vi "Core Actor - CLOSE - External Queues_Notifiers.vi"(8 "error in (no error)":errorcluster, 11 "Child_4_Class in":refnum<class "Logging_Class.lvclass">) -> (0 "error out":errorcluster, 3 "Child_4_Class out":refnum<class "Logging_Class.lvclass">)   [LabVIEW 2023, in "Logging.lvlib" / "Logging_Class.lvclass"]
uses:
  Logging_Class.lvclass
  Abstraction_Interface_Class/Abstraction_Interface_Class.lvclass
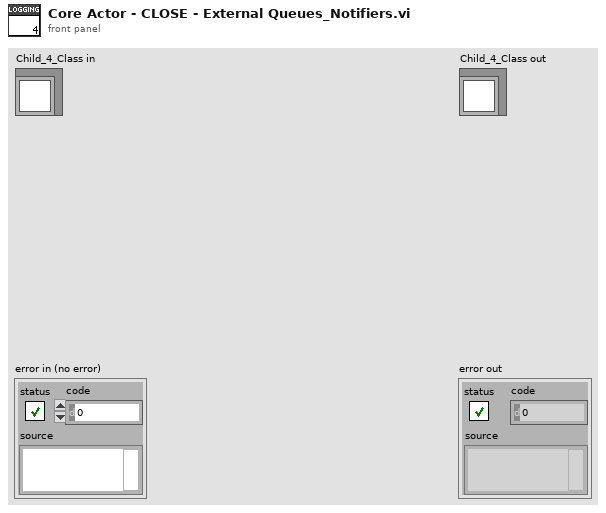
[diagram p1: front panel]
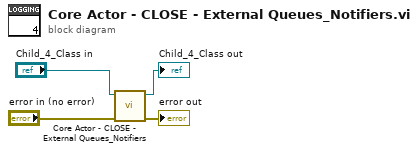
[diagram p0: block diagram]
diagram:
  n1 = call-parent "Core Actor - CLOSE - External Queues_Notifiers.vi"("error in (no error)"="error in (no error)", "Interface_Class in"="Child_4_Class in") -> ("error out"=→"error out":errorcluster, "Interface_Class out"=→"Child_4_Class out":refnum<class "Logging_Class.lvclass">)  [unwired: 8 in]
